vi "Write Single Digital Port.vi"(8 "error in (no error)":errorcluster, 9 "Pin State":bool, 10 "Pin Number":T1(ring), 11 "VISA resource name":refnum<visa-resource-name>) -> (0 "error out":errorcluster, 3 "VISA resource name out":refnum<visa-resource-name>)   [LabVIEW 2020, in "BDAQ-6104.lvlib"]
uses:
  <instrlib>/BDAQ-6104/BDAQ-6104.lvlib
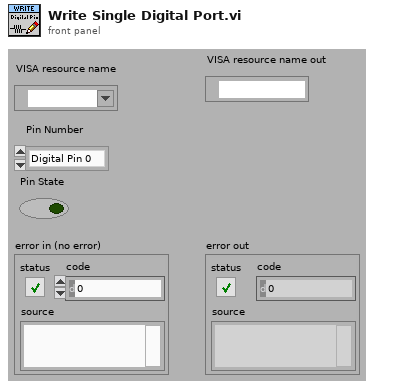
[diagram p1: front panel]
types:
  T1 = enum16{"Digital Pin 0", "Digital Pin 1", "Digital Pin 2", "Digital Pin 3"}
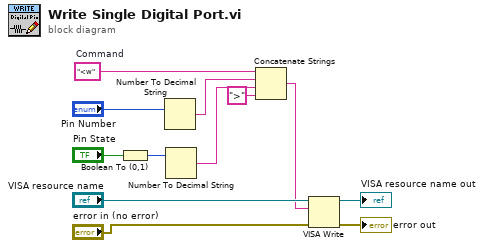
[diagram p0: block diagram]
diagram:
  w8 = "<w"  # Command
  n1 = Boolean To (0,1)(Boolean="Pin State") -> (0, 1=w9:i16)
  n2 = Number To Decimal String(number="Pin Number") -> (decimal integer string=w6:string)  [unwired: 1 in]
  n3 = Number To Decimal String(number=w9) -> (decimal integer string=w5:string)  [unwired: 1 in]
  n4 = Concatenate Strings(w8, w6, w5, ">" ("string")) -> (w3:string)
  n5 = VISA Write(VISA resource name="VISA resource name", write buffer=w3, error in (no error)="error in (no error)") -> (VISA resource name out=→"VISA resource name out":refnum<visa-resource-name>, error out=→"error out":errorcluster)  [unwired: 1 out]
